vi "Z Test.vi"(6 "alternative hypothesis":i32(ring) items=["mean(pop) != mean"=0, "mean(pop) > mean"=1, "mean(pop) < mean"=-1], 8 "std":dbl=1.0, 9 "significance level":dbl=0.05, 10 "mean":dbl, 11 "sample set":dbl[](array[numeric])) -> (0 "error":i32, 1 "confidence interval":cluster{"low":dbl, "high":dbl}={"low"=0.8260722090132093, "high"=0.8260722090132093} {"high" format="%.6g"; "low" format="%.6g"}, 2 "p value":dbl=0.05 format="%.6g", 3 "reject null hypothesis":bool, 4 "z test info":T1 {"sample z value" format="%_6g"; "z value" format="%_6g"; "sample se mean" format="%_6g"; "sample std" format="%_6g"; "sample mean" format="%_6g"})   [LabVIEW 2017, in "NI_Gmath.lvlib"]
doc: "Tests hypotheses about the <B>mean</B> of a population whose distribution is at least approximately normal and whose variance is known."
uses:
  NI_Gmath.lvlib
  st_z_control.ctl
  NI_AALBase.lvlib
panel:
  # "Z Test\n(single sample set)"
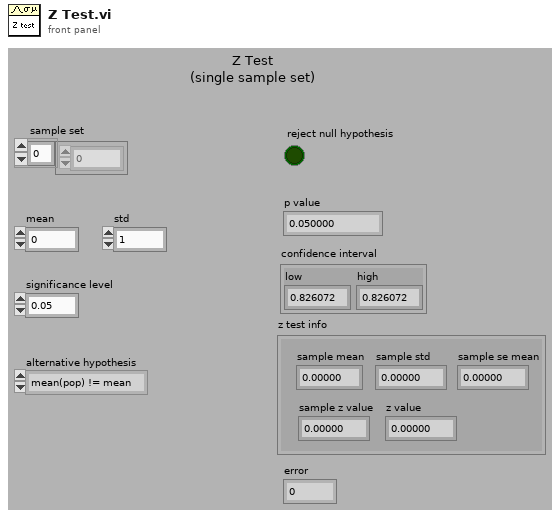
[diagram p1: front panel]
types:
  T1 = typedef "NI_Gmath.lvlib/st_z_control.ctl" = cluster{"sample mean":dbl, "sample std":dbl, "sample se mean":dbl, "sample z value":dbl, "z value":dbl}
  T2 = cluster{"sample mean":dbl, "sample std":dbl, "sample se mean":dbl, "z value":dbl, "sample z value":dbl}
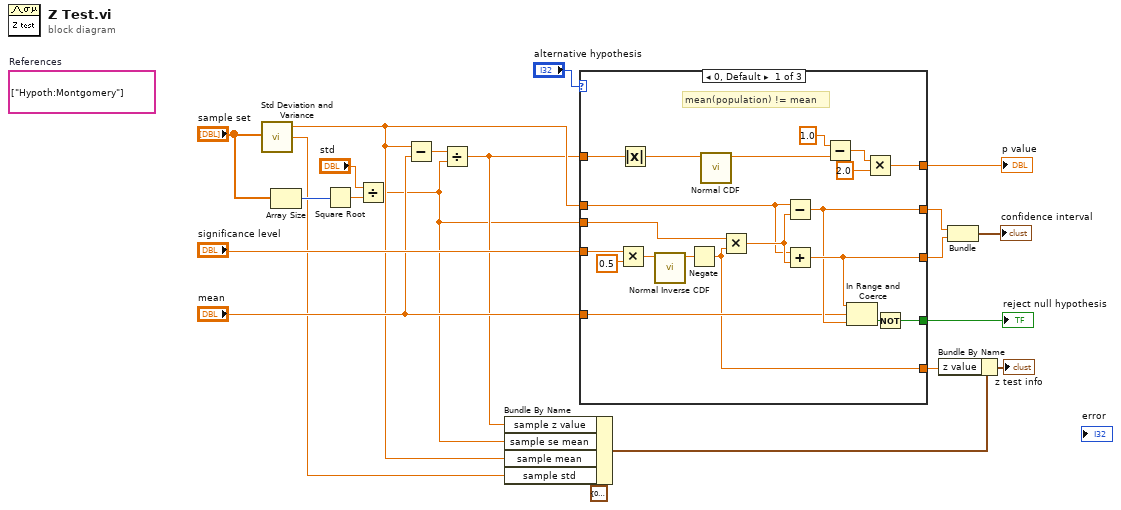
[diagram p0: block diagram]
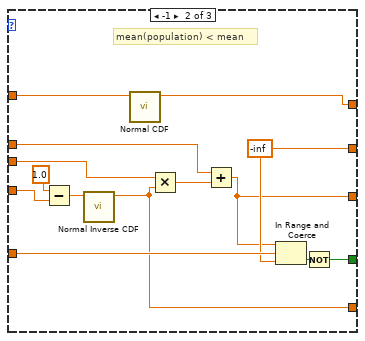
[diagram p2: hidden frame]
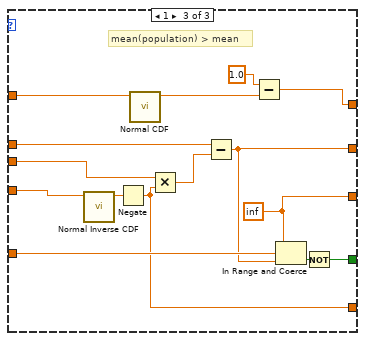
[diagram p3: hidden frame]
diagram:
  (unwired) string[] ["Hypoth:Montgomery"]  # References
  n1 = call "Std Deviation and Variance.vi"("X"="sample set") -> ("mean"=w8:dbl, "standard deviation"=w1:dbl)  [unwired: 1 in, 1 out]
  n2 = Array Size(array="sample set") -> (size(s)=w10:i32)
  n3 = Square Root(x=w10) -> (sqrt(x)=w11:dbl)
  n4 = Divide(x="std", y=w11) -> (x/y=w6:dbl)
  n5 = Subtract(x=w8, y="mean") -> (x-y=w20:dbl)
  n6 = Divide(x=w20, y=w6) -> (x/y=w7:dbl)
  n7 = Bundle By Name(cluster=T2 {"sample mean"=0.0, "sample std"=0.0, "sample se mean"=0.0, "z value"=0.0, "sample z value"=0.0} ("t test info"), "sample z value"=w7, "sample se mean"=w6, "sample mean"=w8, "sample std"=w1) -> (w3:T2)
  n8 = case shown="0, Default" "alternative hypothesis" {
    tunnel: "significance level" -> [w40 w48 w62]
    tunnel: w6 -> [w39 w55 w70]
    tunnel: [w35 w43 w59] -> w17
    tunnel: [w34 w44 w60] -> w16
    tunnel: [w32 w52 w67] -> w15
    tunnel: "mean" -> [w31 w51 w66]
    tunnel: w8 -> [w30 w50 w61]
    tunnel: w7 -> [w29 w45 w65]
    tunnel: [w24 w42 w58] -> w12
    tunnel: [w23 w46 w56] -> w5
    frame 0, Default {
      # "mean(population) != mean"
      n9 = Multiply(x=w40, y=0.5) -> (x*y=w36:dbl)
      n10 = Absolute Value(x=w29) -> (abs(x)=w22:dbl)
      n11 = call "Normal Inverse CDF.vi"("cdf(x)"=w36) -> ("x"=w37:dbl)  [unwired: 9 in, 1 out]
      n12 = Negate(x=w37) -> (-x=w23:dbl)
      n13 = call "Normal CDF.vi"("x"=w22) -> ("cdf(x)"=w27:dbl)  [unwired: 9 in, 1 out]
      n14 = Multiply(x=w39, y=w23) -> (x*y=w38:dbl)
      n15 = Subtract(x=w30, y=w38) -> (x-y=w34:dbl)
      n16 = Add(x=w30, y=w38) -> (x+y=w35:dbl)
      n17 = Subtract(x=1.0, y=w27) -> (x-y=w25:dbl)
      n18 = In Range and Coerce(upper limit=w35, x=w31, lower limit=w34) -> (In Range?=w33:bool)  [unwired: 1 out]
      n19 = Multiply(x=w25, y=2.0) -> (x*y=w24:dbl)
      n20 = Not(x=w33) -> (.not. x?=w32:bool)
    }
    frame -1 {
      w44 = -inf ("lower limit")
      # "mean(population) < mean"
      n21 = Subtract(x=1.0, y=w48) -> (x-y=w47:dbl)
      n22 = call "Normal Inverse CDF.vi"("cdf(x)"=w47) -> ("x"=w46:dbl)  [unwired: 9 in, 1 out]
      n23 = call "Normal CDF.vi"("x"=w45) -> ("cdf(x)"=w42:dbl)  [unwired: 9 in, 1 out]
      n24 = Multiply(x=w55, y=w46) -> (x*y=w54:dbl)
      n25 = Add(x=w50, y=w54) -> (x+y=w43:dbl)
      n26 = In Range and Coerce(upper limit=w43, x=w51, lower limit=w44) -> (In Range?=w53:bool)  [unwired: 1 out]
      n27 = Not(x=w53) -> (.not. x?=w52:bool)
    }
    frame 1 {
      w59 = inf
      # "mean(population) > mean"
      n28 = call "Normal Inverse CDF.vi"("cdf(x)"=w62) -> ("x"=w57:dbl)  [unwired: 9 in, 1 out]
      n29 = Negate(x=w57) -> (-x=w56:dbl)
      n30 = call "Normal CDF.vi"("x"=w65) -> ("cdf(x)"=w63:dbl)  [unwired: 9 in, 1 out]
      n31 = Multiply(x=w70, y=w56) -> (x*y=w69:dbl)
      n32 = Subtract(x=w61, y=w69) -> (x-y=w60:dbl)
      n33 = Subtract(x=1.0, y=w63) -> (x-y=w58:dbl)
      n34 = In Range and Coerce(upper limit=w59, x=w66, lower limit=w60) -> (In Range?=w68:bool)  [unwired: 1 out]
      n35 = Not(x=w68) -> (.not. x?=w67:bool)
    }
  }
  "reject null hypothesis" <- w15
  "p value" <- w12
  n36 = Bundle By Name(cluster=w3, "z value"=w5) -> (→"z test info":T2)
  n37 = Bundle("lower limit"=w16, w17) -> (→"confidence interval":cluster{"lower limit":dbl, dbl})  [unwired: 1 in]
